vi "Unlock.vi"(8 "error in (no error)":errorcluster, 11 "Timed Door in":refnum<class "Timed Door.lvclass">) -> (0 "error out":errorcluster, 3 "Timed Door out":refnum<class "Timed Door.lvclass">)   [LabVIEW 2018, in "Timed Door.lvclass"]
uses:
  Timed Door.lvclass
  Timed Door.lvclass/Timed Door.ctl
  Timer/Timer.lvclass
  Timer/Timer.lvclass/Timer.ctl
  Get Door.vi
  Set Door.vi
  Timer/Get Target Time Elapsed Event.vi
  Set Timer DVR.vi
  Set Target Time Elapsed Event.vi
  Set Alarm DVR.vi
  Door/Door.lvclass
  Alarm/Alarm.lvclass
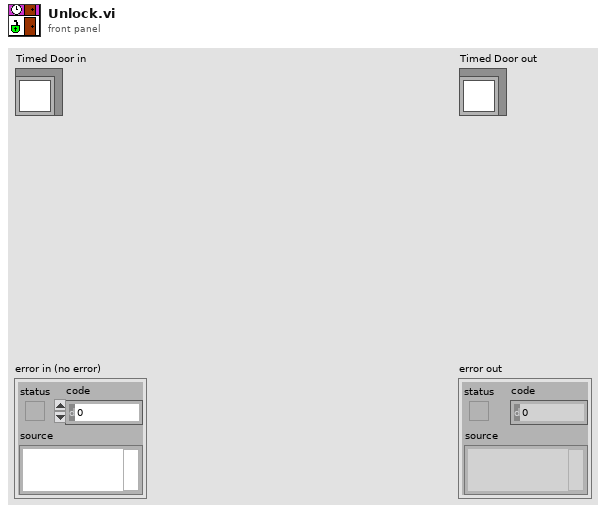
[diagram p1: front panel]
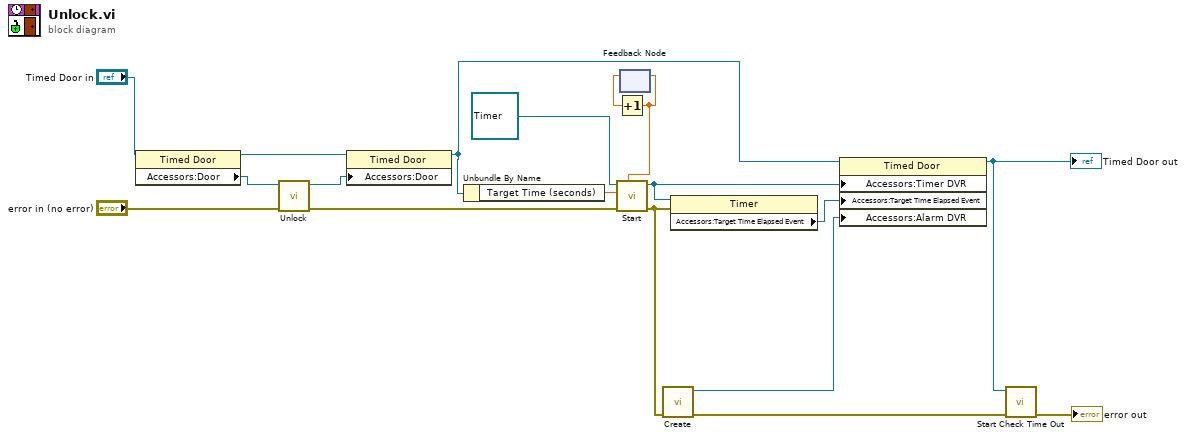
[diagram p0: block diagram]
diagram:
  n1 = property class="Timed Door"(reference="Timed Door in") -> (reference out=w2:refnum<class "Timed Door.lvclass">, "Accessors:Door"=w4:refnum<class "Door.lvclass">)  [unwired: 1 in, 1 out]
  n2 = call-dynamic "Unlock.vi"("error in (no error)"="error in (no error)", "Door in"=w4) -> ("error out"=w15:errorcluster, "Door out"=w3:refnum<class "Door.lvclass">)  [unwired: 8 in]
  n3 = property class="Timed Door"(reference=w2, "Accessors:Door"=w3) -> (reference out=w1:refnum<class "Timed Door.lvclass">)  [unwired: 1 in, 1 out]
  n4 = Unbundle By Name(w1) -> ("Target Time (seconds)"=w17:dbl)
  n5 = feedback #1() -> (w7:dbl)  [unwired: 1 in]
  n6 = Increment(x=w7) -> (x+1=w6:dbl)
  n7 = call-dynamic "Start.vi"("Timer ID"=w6, "error in (no error)"=w15, "Target Time (seconds)"=w17, "Timer in"=refnum<class "Timer.lvclass"> refnum) -> ("error out"=w10:errorcluster, "Timer DVR"=w9:refnum<data-value>)  [unwired: 6 in]
  n8 = feedback-in #1(w6) -> ()
  n9 = call "Create.vi"("error in (no error)"=w10) -> ("error out"=w11:errorcluster, "Alarm DVR"=w13:refnum<data-value>)  [unwired: 9 in]
  n10 = property class="Timer"(reference=w9, error in=w10) -> ("Accessors:Target Time Elapsed Event"=w8:refnum<user-event>)  [unwired: 2 out]
  n11 = property class="Timed Door"(reference=w1, "Accessors:Timer DVR"=w9, "Accessors:Target Time Elapsed Event"=w8, "Accessors:Alarm DVR"=w13) -> (reference out=w12:refnum<class "Timed Door.lvclass">)  [unwired: 1 in, 1 out]
  "Timed Door out" <- w12
  n12 = call "Start Check Time Out.vi"("error in (no error)"=w11, "Timed Door in"=w12) -> ("error out"=→"error out":errorcluster)  [unwired: 9 in]
